vi "State_SET.vi"(8 "error in":errorcluster, 10 "state":T1, 11 "tcp server in":refnum<class "RT FlexRIO Server TCP.lvclass">) -> (0 "error out":errorcluster, 3 "tcp server out":refnum<class "RT FlexRIO Server TCP.lvclass">)   [LabVIEW 2017, in "RT FlexRIO Server TCP.lvclass"]
uses:
  RT FlexRIO Server TCP.lvclass
  Public/State.ctl
  RT FlexRIO Server TCP.lvclass/RT FlexRIO Server TCP.ctl
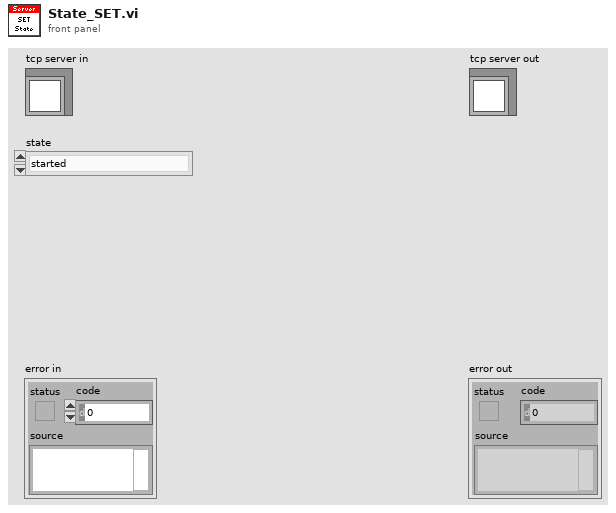
[diagram p1: front panel]
types:
  T1 = typedef "RT FlexRIO Server TCP.lvclass/State.ctl" = enum16{"started", "connected", "stopped"}
  T2 = typedef "RT FlexRIO Server TCP.lvclass/SessionData.ctl" = cluster{"listener":refnum<k5>, "connection":refnum<k5>, "state":T3, "incoming":refnum<queue>, "outgoing":refnum<queue>, "state request":refnum<user-event>, "state changed":refnum<user-event>}
  T3 = typedef "RT FlexRIO Server TCP.lvclass/connection state.ctl" = enum16{"started", "connected", "stopped"}
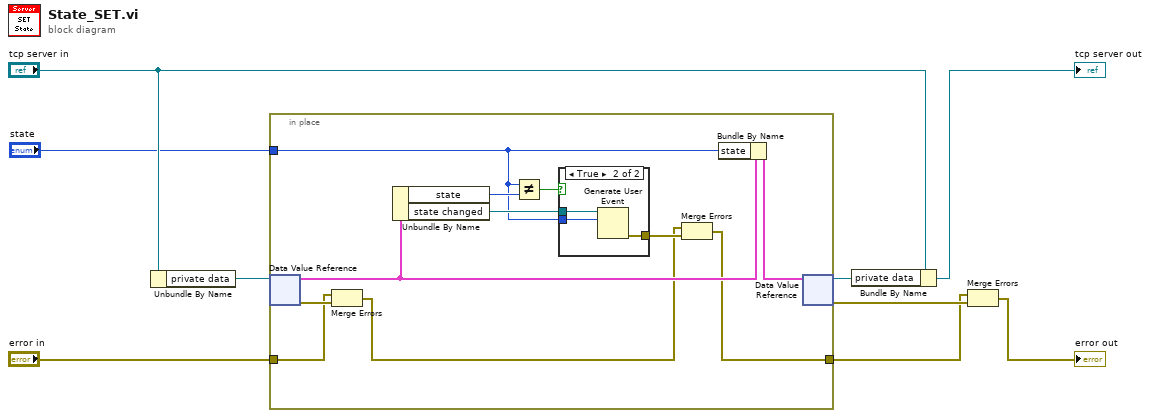
[diagram p0: block diagram]
diagram:
  n1 = Unbundle By Name("tcp server in") -> ("private data"=w4:refnum<data-value>)
  n2 = in-place {
    in-place-border: "error in" -> [w19]
    in-place-border: [w10] -> w2
    in-place-border: "state" -> [w14]
    n3 = in-place-dvr #1(w4) -> (w13:T2, w20:errorcluster)
    n4 = Merge Errors(w19, w20) -> (w11:errorcluster)
    n5 = Unbundle By Name(w13) -> ("state"=w17:T3, "state changed"=w15:refnum<user-event>)
    n6 = Not Equal?(x=w14, y=w17) -> (x != y?=w16:bool)
    n7 = case shown="True" w16 {
      tunnel: w15 -> [_ w23]
      tunnel: w14 -> [_ w22]
      tunnel: [_ w21] -> w12
      frame False {
      }
      frame True {
        n8 = Generate User Event(user event=w23, event data cluster=w22) -> (error out=w21:errorcluster)  [unwired: 2 in, 1 out]
      }
    }
    n9 = Merge Errors(w11, w12) -> (w10:errorcluster)
    n10 = Bundle By Name(cluster=w13, "state"=w14) -> (w18:T2)
    n11 = in-place-dvr #1(w18) -> (w1:refnum<data-value>, w3:errorcluster)
  }
  n12 = Bundle By Name(cluster="tcp server in", "private data"=w1) -> (→"tcp server out":refnum<class "RT FlexRIO Server TCP.lvclass">)
  n13 = Merge Errors(w2, w3) -> (→"error out":errorcluster)
